vi "32ScanBarcodeJW.vi"(4 "no check?":bool, 6 "条码长度1":i32=6, 7 "总数1":i32=6) -> (0 "电子表格字符串":string, 1 "Barcodes out":string[](array[string]), 2 "canceled":bool, 3 "PF":bool[](array[boolean]))   [LabVIEW 2018]
uses:
  Global.vi
panel:
  in  "退出程序":bool
  in  "条码数量":string
  in  "条码长度":string
  in  "重置":bool
  out "长度":i32
  out "数组":string[](array[string])
  out "Length 2":i32
  in  "Barcode 32":string
  in  "Barcode31":string
  in  "Barcode 30":string
  in  "Barcode 29":string
  in  "Barcode 28":string
  in  "Barcode 27":string
  in  "Barcode 26":string
  in  "Barcode 25":string
  in  "Barcode 24":string
  in  "Barcode23":string
  in  "Barcode22":string
  in  "Barcode 21":string
  in  "Barcode 20":string
  in  "Barcode 19":string
  in  "Barcode 18":string
  in  "Barcode17":string
  in  "Barcode 16":string
  in  "Barcode 15":string
  in  "Barcode 14":string
  in  "Barcode 13":string
  in  "Barcode 12":string
  in  "Barcode 11":string
  in  "Barcode 10":string
  in  "Barcode 9":string
  in  "Barcode 8":string
  in  "Barcode 7":string
  in  "Barcode 6":string
  in  "Barcode 5":string
  in  "Barcode 4":string
  in  "Barcode 3":string
  in  "Barcode 2":string
  in  "Barcode 1":string
  out "barcode refrencesd":refnum<vi>[](array[refnum])
  in  "esc":bool
  in  "OK":bool
  # "请使用扫描枪扫描条码或二维码!放弃请按\"ESC\"键!"
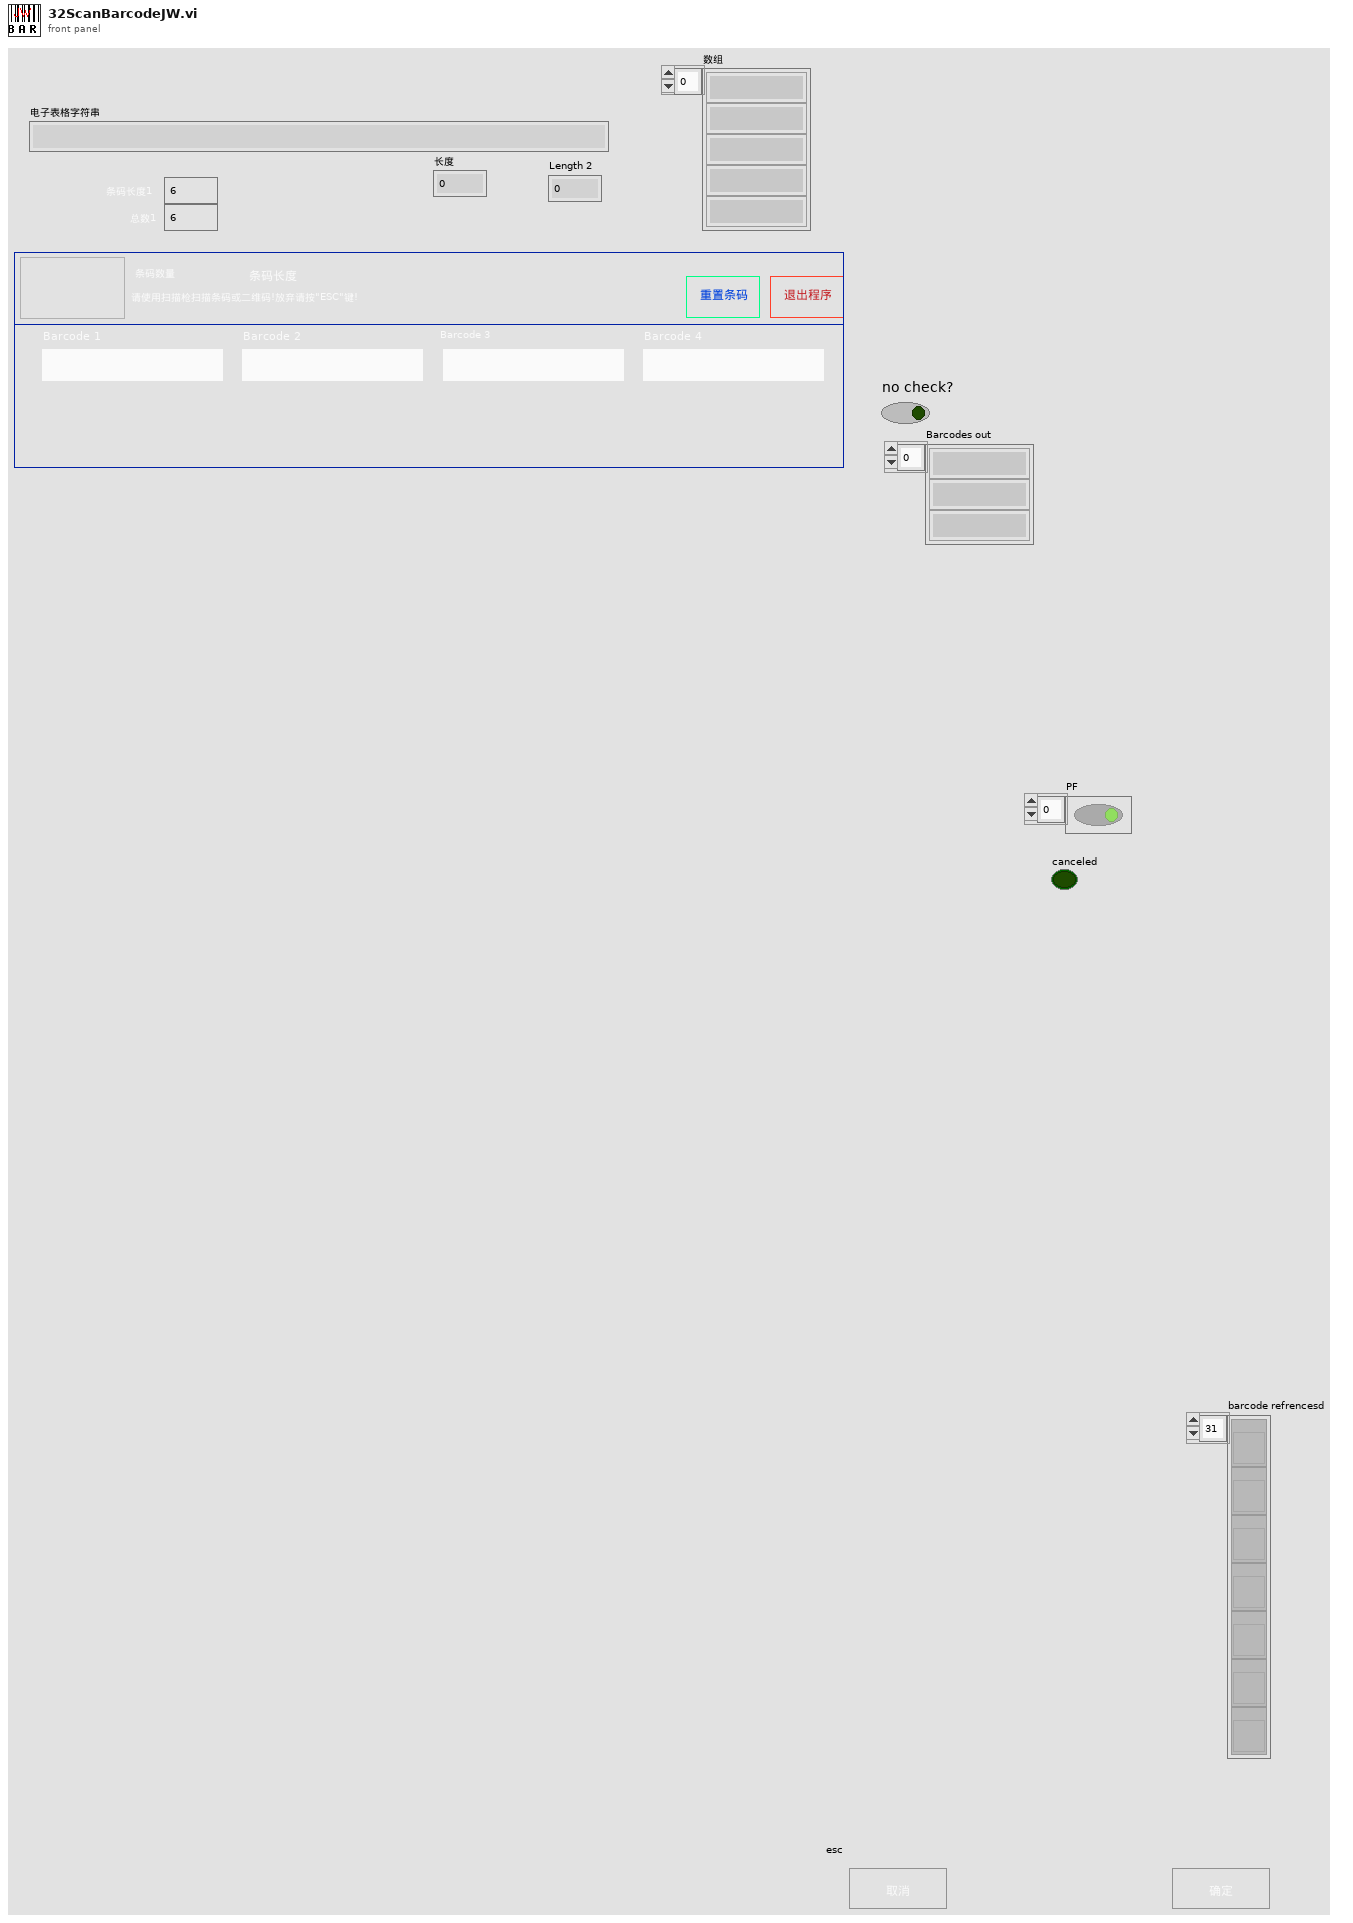
[diagram p1: front panel]
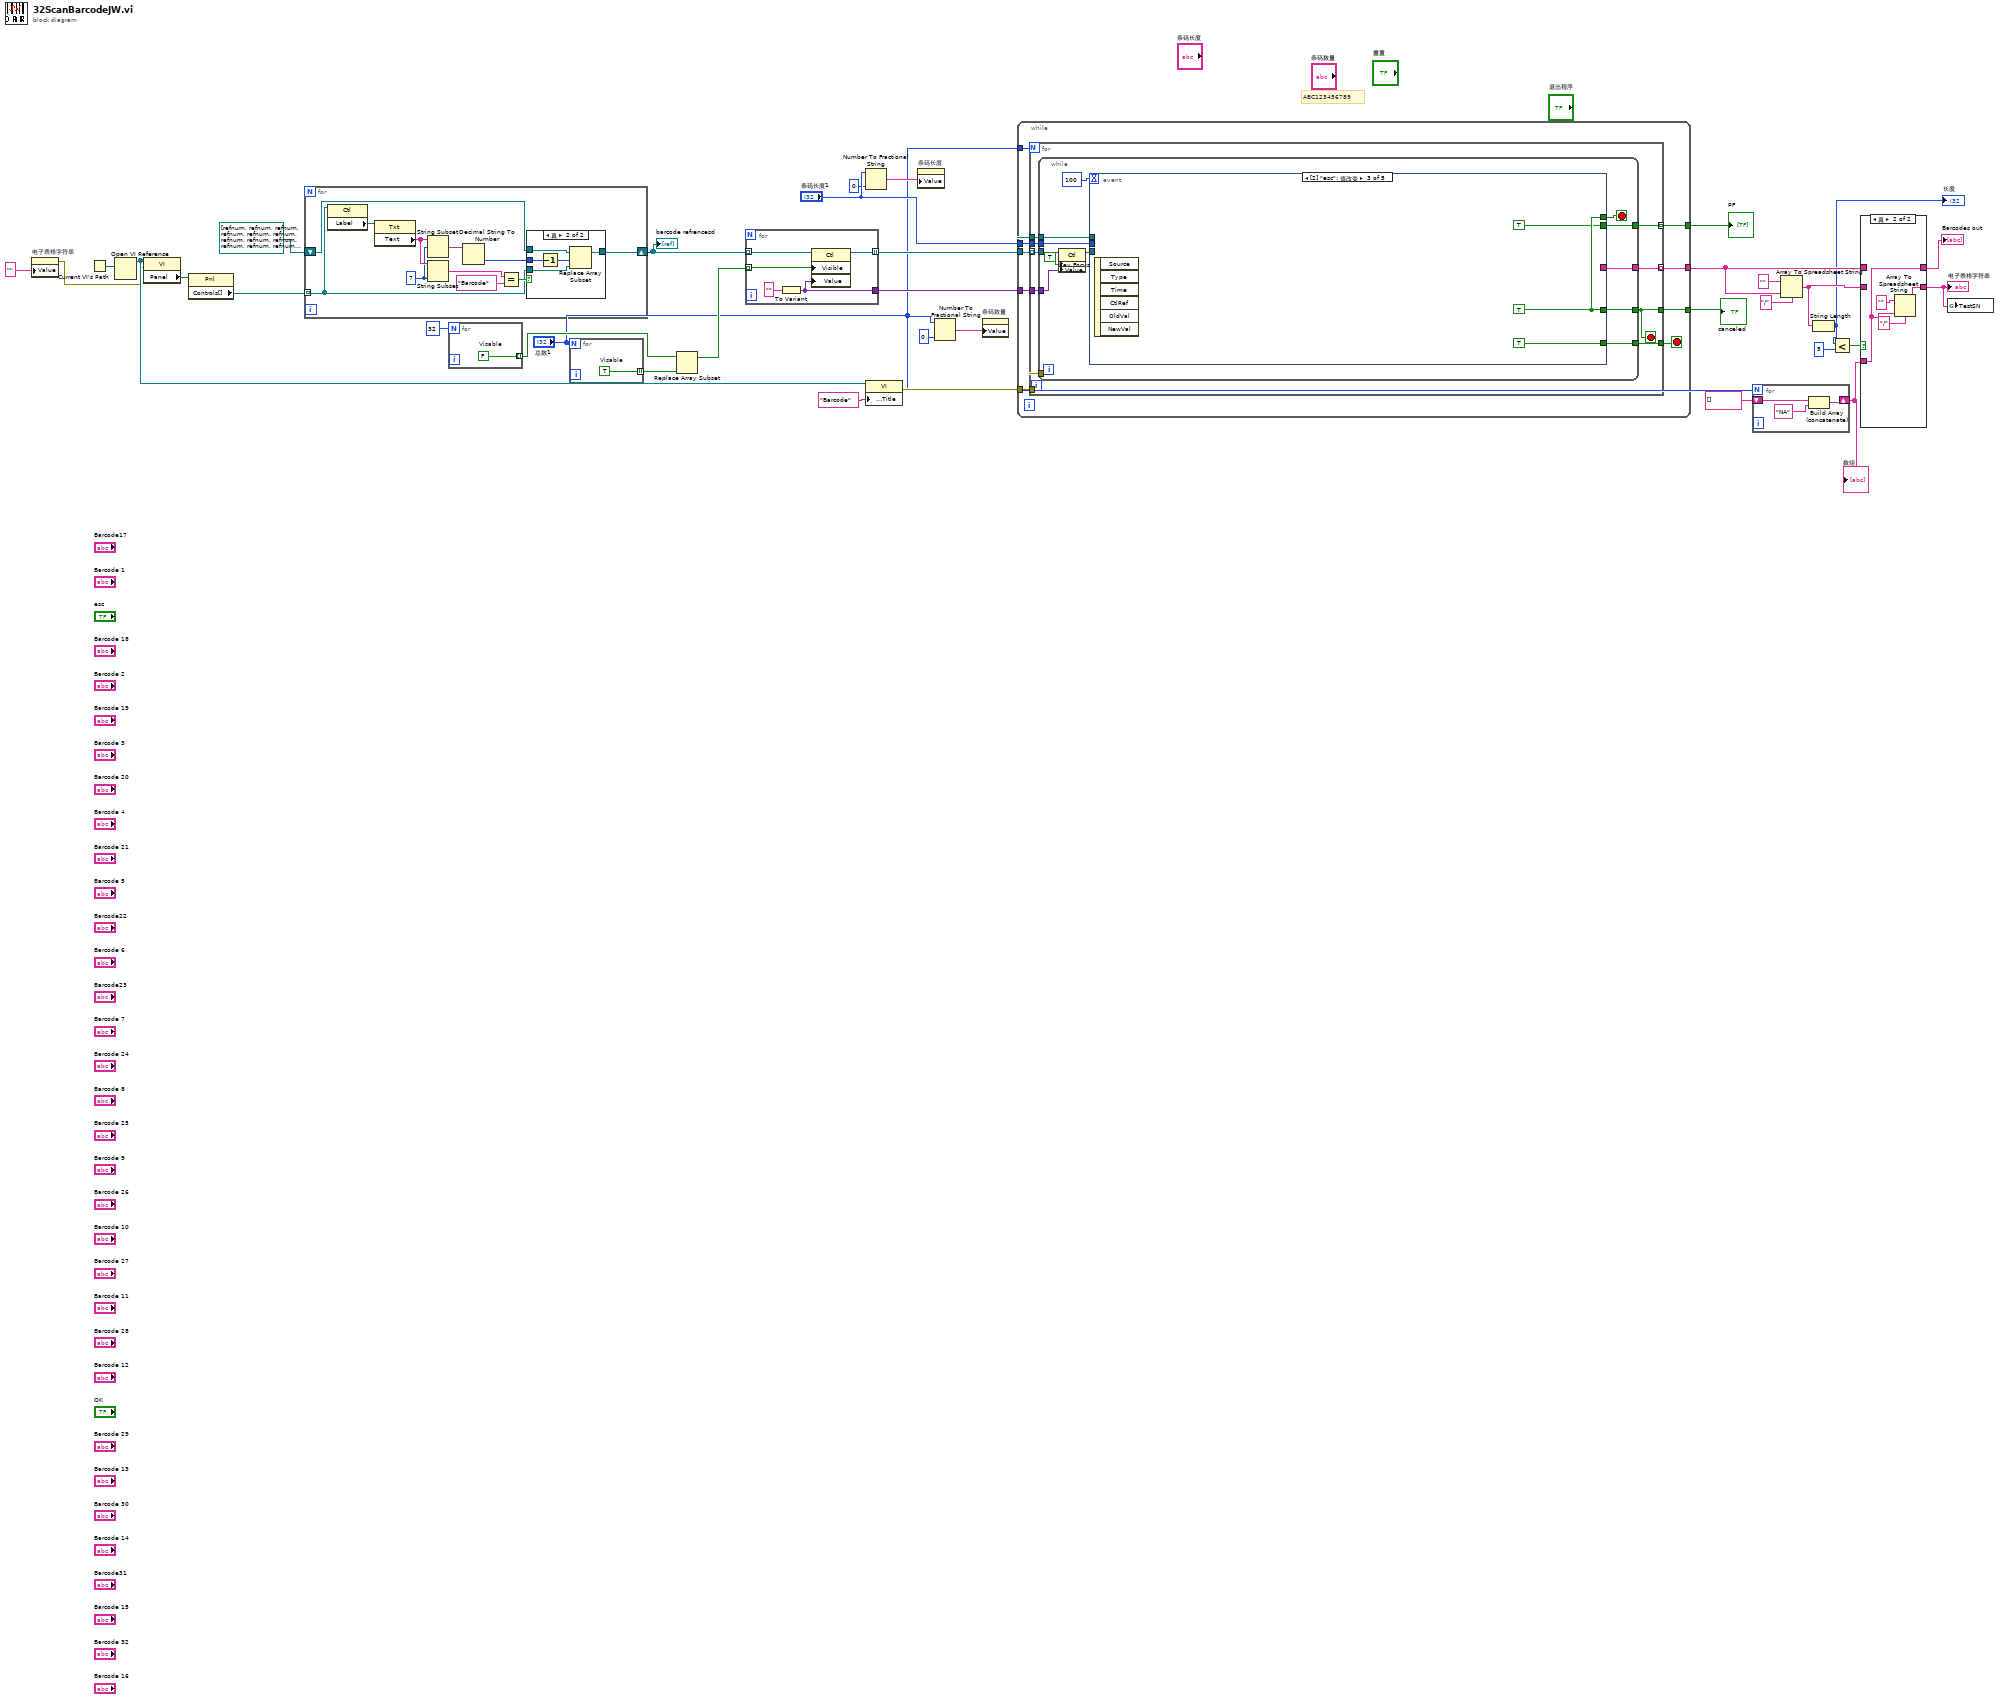
[diagram p0: block diagram]
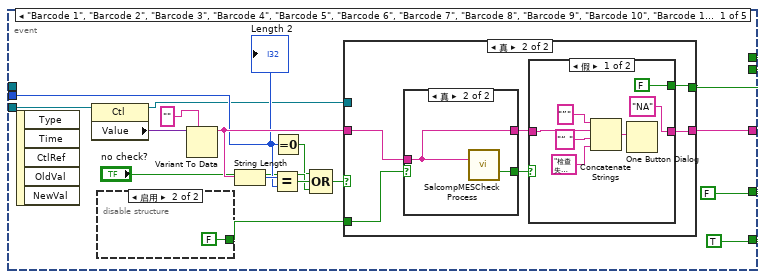
[diagram p2: hidden frame]
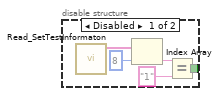
[diagram p3: hidden frame]
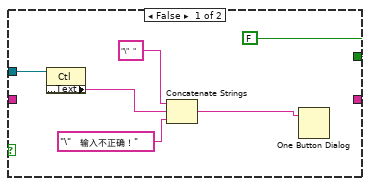
[diagram p4: hidden frame]
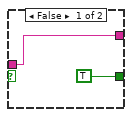
[diagram p5: hidden frame]
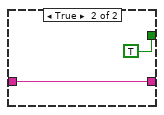
[diagram p6: hidden frame]
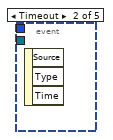
[diagram p7: hidden frame]
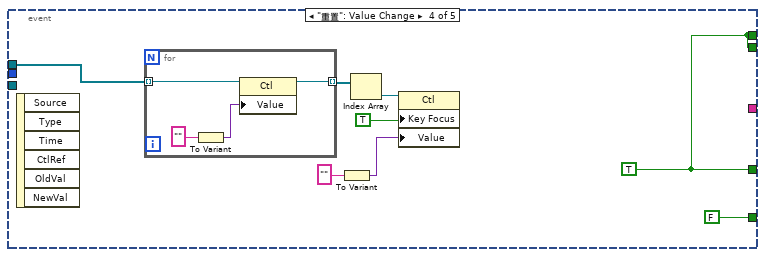
[diagram p8: hidden frame]
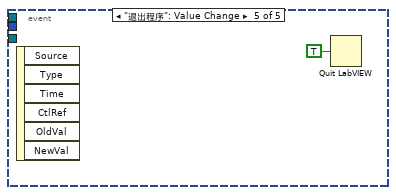
[diagram p9: hidden frame]
diagram:
  # "ABC123456789"
  n1 = property on="电子表格字符串" class="Str"("Value"="") -> (error out=w10:errorcluster)  [unwired: 2 in, 1 out]
  n2 = Current VI's Path() -> (path=w35:path)
  n3 = Open VI Reference(vi path=w35) -> (vi reference=w32:refnum<vi>)  [unwired: 2 in, 4 out]
  n4 = property class="VI"(reference=w32, error in=w10) -> ("Panel"=w31:refnum<vi>)  [unwired: 2 out]
  n5 = property class="Pnl"(reference=w31) -> ("Controls[]"=w30:refnum<vi>[])  [unwired: 1 in, 2 out]
  n6 = for {
    tunnel: w30 -> [w36] mode=indexing
    shift-right: [w45] -> w29
    shift-left: refnum<vi>[] [refnum, refnum, refnum, refnum, refnum, refnum, refnum, refnum, refnum, refnum, refnum, refnum, refnum, refnum, refnum, refnum, refnum, refnum, refnum, refnum, refnum, refnum, refnum, refnum, refnum, refnum, refnum, refnum, refnum, refnum, refnum, refnum] ("barcode refrencesd 2") -> [w46]
    w39 = 7 ("长度（剩余）")
    n7 = property class="Ctl"(reference=w36) -> ("Label"=w44:refnum<vi>)  [unwired: 1 in, 2 out]
    n8 = property class="Txt"(reference=w44) -> ("Text"=w40:string)  [unwired: 1 in, 2 out]
    n9 = String Subset(string=w40, offset (0)=w39) -> (substring=w38:string)  [unwired: 1 out]
    n10 = String Subset(string=w40, length (rest)=w39) -> (substring=w42:string)  [unwired: 1 out]
    n11 = Decimal String To Number(string=w38) -> (number=w37:i32)  [unwired: 3 out]
    n12 = Equal?(x=w42, y="Barcode") -> (x = y?=w41:bool)
    n13 = case shown="真" w41 {
      tunnel: w46 -> [w47 w52]
      tunnel: [w47 w51] -> w45
      tunnel: w37 -> [_ w50]
      tunnel: w36 -> [_ w48]
      frame False {
      }
      frame True {
        n14 = Decrement(x=w50) -> (x-1=w49:i32)
        n15 = Replace Array Subset(array=w52, new element=w48, index=w49) -> (w51:refnum<vi>[])
      }
    }
  }
  "barcode refrencesd" <- w29
  n16 = for {
    N: 32 -> [_]
    tunnel: [w53] -> w28 mode=indexing
    w53 = FALSE  # Visable
  }
  n17 = for {
    N: "总数1" -> [_]
    tunnel: [w54] -> w19 mode=indexing
    w54 = TRUE  # Visable
  }
  n18 = Replace Array Subset(array=w28, new element=w19) -> (w27:bool[])  [unwired: 1 in]
  n19 = for {
    tunnel: w29 -> [w59] mode=indexing
    tunnel: w27 -> [w58] mode=indexing
    tunnel: [w56] -> w7 mode=indexing
    tunnel: [w55] -> w23
    n20 = To Variant(anything="") -> (Variant=w55:variant)
    n21 = property class="Ctl"(reference=w59, "Visible"=w58, "Value"=w55) -> (reference out=w56:refnum<vi>)  [unwired: 1 in, 1 out]
  }
  n22 = Number To Fractional String(number="条码长度1", precision (6)=i16 0 ("精度(6)")) -> (F-format string=w4:string)  [unwired: 2 in]
  n23 = property class="VI"(reference=w32, "Front Panel.Title"="Barcode" ("前面板窗口:标题")) -> (error out=w34:errorcluster)  [unwired: 1 in, 1 out]
  n24 = property on="条码长度" class="Str"("Value"=w4) -> ()  [unwired: 2 in, 2 out]
  n25 = Number To Fractional String(number="总数1", precision (6)=i16 0 ("精度(6)")) -> (F-format string=w1:string)  [unwired: 2 in]
  n26 = property on="条码数量" class="Str"("Value"=w1) -> ()  [unwired: 2 in, 2 out]
  n27 = while {
    tunnel: w34 -> [w68]
    tunnel: [w67] -> w24
    tunnel: w23 -> [w66]
    tunnel: [w65] -> w22
    tunnel: [w64] -> w15
    tunnel: "条码长度1" -> [w63]
    tunnel: "总数1" -> [w62]
    tunnel: w7 -> [w61]
    stop <- w60 stop-if-true
    n28 = for {
      N: w62 -> [_]
      tunnel: w68 -> [w77]
      tunnel: [w76] -> w64 mode=indexing
      tunnel: [w75] -> w67 mode=indexing
      tunnel: w61 -> [w74] mode=indexing
      tunnel: w63 -> [w73]
      tunnel: w66 -> [w72]
      tunnel: [w71] -> w65
      tunnel: w61 -> [w70]
      tunnel: [w69] -> w60
      stop <- w71 stop-if-true
      n29 = while {
        tunnel: [w85] -> w75
        tunnel: [w89] -> w76
        tunnel: w77 -> [_]
        tunnel: w74 -> [w81]
        tunnel: w73 -> [w86]
        tunnel: w72 -> [w80]
        tunnel: [w82] -> w71
        tunnel: w70 -> [w79]
        tunnel: [w78] -> w69
        stop <- w83 stop-if-true
        n30 = property class="Ctl"(reference=w81, "Key Focus"=TRUE ("键选中"), "Value"=w80) -> (reference out=w87:refnum<vi>)  [unwired: 1 in, 1 out]
        n31 = event shown="[2] \"esc\": 值改变" {
          selector: _ -> [_ _ _ _ _]
          dyn-events: _ -> [_ _ _ _ _]
          timeout: 100 -> [_ _ _ _ _]
          tunnel: [w104 _ _ _ _] -> w89
          tunnel: w87 -> [w103 _ _ _ _]
          tunnel: w86 -> [w99 _ _ _ _]
          tunnel: [w98 _ w139 w141 _] -> w83
          tunnel: [w98 _ TRUE w141 _] -> w85
          tunnel: [FALSE _ w139 w141 _] -> w82
          tunnel: w79 -> [_ _ _ w147 _]
          tunnel: [TRUE _ TRUE FALSE _] -> w78
          event "Barcode 1", "Barcode 2", "Barcode 3", "Barcode 4", "Barcode 5", "Barcode 6", "Barcode 7", "Barcode 8", "Barcode 9", "Barcode 10", "Barcode 11", "Barcode 12", "Barcode 13", "Barcode 14", "Barcode 15", "Barcode 16", "Barcode17", "Barcode 18", "Barcode 19", "Barcode 20", "Barcode 21", "Barcode22", "Barcode23", "Barcode 24", "Barcode 26", "Barcode 25", "Barcode 27", "Barcode 28", "Barcode 29", "Barcode 30", "Barcode31", "Barcode 32": Value Change {
            n32 = event-data() -> ()  [unwired: 6 out]
            n33 = property class="Ctl"(reference=w103) -> (reference out=w93:refnum<vi>, "Value"=w102:variant)  [unwired: 1 in, 1 out]
            n34 = disable-structure shown="启用" {
              disable-tunnel: [w106 FALSE] -> w91
              frame Disabled {
                n35 = call "Read_SetTestInformaton.vi"() -> ("数组 2"=w110:string[])  [unwired: 7 in, 4 out]
                n36 = Index Array(array=w110, index=8 ("索引")) -> (element=w109:string)
                n37 = Equal?(x=w109, y="1") -> (x = y?=w106:bool)
              }
              frame Enabled {
              }
            }
            n38 = Variant To Data(type="", Variant=w102) -> (data=w100:string)  [unwired: 1 in, 1 out]
            n39 = String Length(string=w100) -> (length=w105:i32)
            n40 = Equal?(x=w105, y=w99) -> (x = y?=w97:bool)
            n41 = Equal To 0?(x=w99) -> (x = 0?=w94:bool)
            n42 = Compound Arithmetic op=OR(w94, w97, "no check?") -> (w96:bool)
            n43 = case shown="真" w96 {
              tunnel: [FALSE w123] -> w98
              tunnel: w100 -> [_ w121]
              tunnel: [_ w118] -> w104
              tunnel: w93 -> [w116 _]
              tunnel: w91 -> [_ w120]
              frame False {
                n44 = property class="Ctl"(reference=w116) -> ("Label.Text"=w115:string)  [unwired: 1 in, 2 out]
                n45 = Concatenate Strings("\"  " ("消息"), w115, "\"   输入不正确！" ("消息")) -> (w114:string)
                n46 = One Button Dialog(message=w114) -> ()  [unwired: 2 out]
              }
              frame True {
                n47 = case shown="真" w120 {
                  tunnel: [TRUE ("CheckRouteForSerialNumber") w127] -> w122
                  tunnel: w121 -> [w124 w126]
                  tunnel: [w124 w126] -> w119
                  frame False {
                  }
                  frame True {
                    n48 = call "SalcompMESCheck Process.vi"("SN"=w126) -> ("CheckRouteForSerialNumber"=w127:bool)  [unwired: 12 in, 2 out]
                  }
                }
                n49 = case shown="假" w122 {
                  tunnel: [FALSE TRUE] -> w123
                  tunnel: w119 -> [w130 w135]
                  tunnel: ["NA" w135] -> w118
                  frame False {
                    n50 = Concatenate Strings("”", w130, "“ ", "检查失败？？？" ("消息")) -> (w133:string)
                    n51 = One Button Dialog(message=w133) -> ()  [unwired: 1 in, 1 out]
                  }
                  frame True {
                  }
                }
              }
            }
            "Length 2" <- w99
          }
          event Timeout {
            n52 = event-data() -> ()  [unwired: 4 out]
          }
          event "esc": Value Change {
            w139 = TRUE
            n53 = event-data() -> ()  [unwired: 7 out]
          }
          event "重置": Value Change {
            w141 = TRUE
            n54 = event-data() -> ()  [unwired: 7 out]
            n55 = for {
              tunnel: w147 -> [w151] mode=indexing
              tunnel: [w149] -> w146 mode=indexing
              n56 = To Variant(anything="") -> (Variant=w148:variant)
              n57 = property class="Ctl"(reference=w151, "Value"=w148) -> (reference out=w149:refnum<vi>)  [unwired: 1 in, 1 out]
            }
            n58 = To Variant(anything="") -> (Variant=w142:variant)
            n59 = Index Array(array=w146) -> (element=w145:refnum<vi>)  [unwired: 1 in]
            n60 = property class="Ctl"(reference=w145, "Key Focus"=TRUE ("键选中"), "Value"=w142) -> ()  [unwired: 1 in, 2 out]
          }
          event "退出程序": Value Change {
            n61 = event-data() -> ()  [unwired: 7 out]
            n62 = Quit LabVIEW(quit? (T)=TRUE ("退出？(T)")) -> ()
          }
        }
      }
    }
  }
  "PF" <- w24
  "canceled" <- w22
  n63 = for {
    N: "总数1" -> [_]
    shift-right: [w153] -> w17
    shift-left: string[] [] -> [w154]
    n64 = Build Array (concatenate)(w154, "NA") -> (w153:string[])
  }
  "数组" <- w17
  n65 = Array To Spreadsheet String(delimiter (Tab)="/" ("分隔符(Tab)"), array=w15, 3:"" ("格式字符串")) -> (spreadsheet string=w13:string)
  n66 = String Length(string=w13) -> (length=w12:i32)
  "长度" <- w12
  n67 = Less?(x=w12, y=5) -> (x < y?=w14:bool)
  n68 = case shown="真" w14 {
    tunnel: [w157 w159] -> w8
    tunnel: w13 -> [w157 _]
    tunnel: w17 -> [_ w158]
    tunnel: [w156 w158] -> w16
    tunnel: w15 -> [w156 _]
    frame False {
    }
    frame True {
      n69 = Array To Spreadsheet String(delimiter (Tab)="/" ("分隔符(Tab)"), array=w158, 3:"" ("格式字符串")) -> (spreadsheet string=w159:string)
    }
  }
  "Barcodes out" <- w16
  "电子表格字符串" <- w8
  n70 = global write "Global.vi" "TestSN"(w8) -> ()
